vi "exercise1.vi"(11 "Acceleration in m/s^2 or g":bool) -> (3 "Data":dbl)   [LabVIEW 2019]
uses:
  <vilib>/DAQmx/read.llb/DAQmx Read (Analog DBL 1Chan 1Samp).vi
  <vilib>/DAQmx/create/channels.llb/DAQmx Create Channel (AI-Voltage-Basic).vi
  <vilib>/DAQmx/miscellaneous.llb/DAQmx Fill In Error Info.vi
panel:
  in  "Numeric":dbl
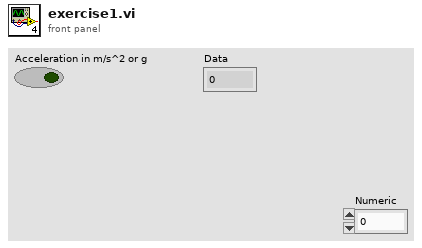
[diagram p1: front panel]
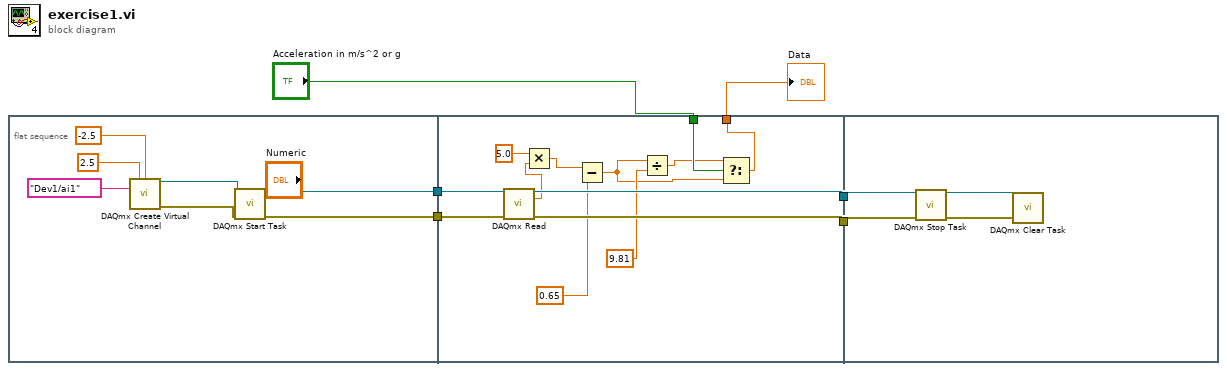
[diagram p0: block diagram]
diagram:
  n1 = flat-sequence {
    tunnel: [w11] -> w6
    tunnel: [w10] -> w5
    tunnel: w6 -> [w26]
    tunnel: w5 -> [w25]
    tunnel: [w20] -> w4
    tunnel: [w24] -> w3
    tunnel: "Acceleration in m/s^2 or g" -> [w23]
    tunnel: [w22] -> w2
    tunnel: w4 -> [w28]
    tunnel: w3 -> [w27]
    frame #0 {
      n2 = call-poly <vilib>:"DAQmx Create Virtual Channel.vi"("maximum value"=2.5, "minimum value"=-2.5, "physical channels"=tag "Dev1/ai1") -> ("task out"=w13:refnum<k21>, "error out"=w12:errorcluster)  [unwired: 11 in]
      n3 = call <vilib>:"DAQmx Start Task.vi"("task/channels in"=w13, "error in"=w12) -> ("task out"=w11:refnum<k21>, "error out"=w10:errorcluster)  [unwired: 12 in]
    }
    frame #1 {
      n4 = call-poly <vilib>:"DAQmx Read.vi"("task/channels in"=w26, "error in"=w25) -> ("task out"=w20:refnum<k21>, "data"=w19:dbl, "error out"=w24:errorcluster)  [unwired: 11 in]
      n5 = Multiply(x=5.0, y=w19) -> (x*y=w21:dbl)
      n6 = Subtract(x=w21, y=0.65) -> (x-y=w14:dbl)
      n7 = Divide(x=w14, y=9.81) -> (x/y=w15:dbl)
      n8 = Select(t=w15, s=w23, f=w14) -> (s? t:f=w22:dbl)
    }
    frame #2 {
      n9 = call <vilib>:"DAQmx Stop Task.vi"("task/channels in"=w28, "error in"=w27) -> ("task out"=w30:refnum<k21>, "error out"=w29:errorcluster)  [unwired: 12 in]
      n10 = call <vilib>:"DAQmx Clear Task.vi"("task in"=w30, "error in"=w29) -> ()  [unwired: 13 in, 1 out]
    }
  }
  "Data" <- w2
